vi "MeasBuilder Path.vi"(11 "error in (no error)":errorcluster) -> (4 "Template":path, 6 "Config":path, 8 "Python File":path, 15 "error out":errorcluster)   [LabVIEW 2021, in "Path Functions.lvlib"]
uses:
  Path Functions.lvlib
  <vilib>/Utility/sysdir.llb/System Directory Type.ctl
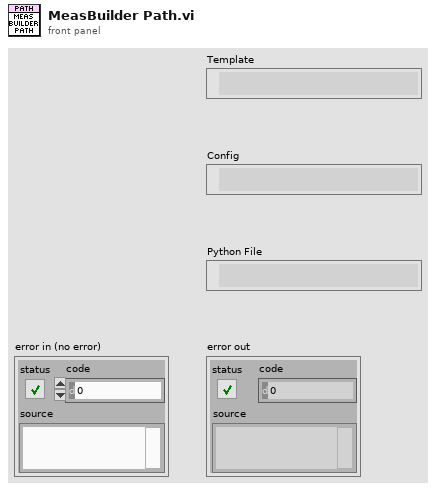
[diagram p1: front panel]
types:
  T1 = typedef "System Directory Type.ctl" = i32
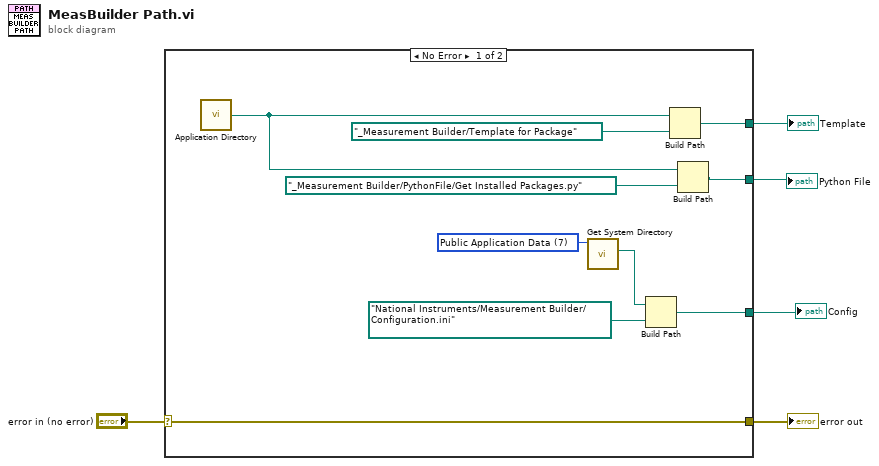
[diagram p0: block diagram]
diagram:
  n1 = case shown="No Error" "error in (no error)" {
    selector: "error in (no error)" -> [w13 w16]
    tunnel: [w14 _] -> w4
    tunnel: [w13 w16] -> w3
    tunnel: [w10 _] -> w2
    tunnel: [w6 _] -> w1
    frame No Error {
      w12 = T1 7 items=["User Home"=0, "User Desktop"=1, "User Documents"=2, "User Application Data"=3, "User Preferences"=4, "User Temporary"=5, "Public Documents"=6, "Public Application Data"=7, "Public Preferences"=8, "Public Cache"=13, "System Core Libraries"=9, "System Installed Libraries"=10, "Application Files"=11, "Boot Volume Root"=12] ("system directory type")
      n2 = call <vilib>:"Application Directory.vi"() -> ("Application Directory"=w7:path)
      n3 = call <vilib>:"Get System Directory.vi"("system directory type"=w12) -> ("system directory"=w11:path)  [unwired: 10 in]
      n4 = Build Path(base path=w11, name or relative path=path "National Instruments/Measurement Builder/Configuration.ini") -> (appended path=w10:path)
      n5 = Build Path(base path=w7, name or relative path=path "_Measurement Builder/Template for Package") -> (appended path=w14:path)
      n6 = Build Path(base path=w7, name or relative path=path "_Measurement Builder/PythonFile/Get Installed Packages.py") -> (appended path=w6:path)
    }
    frame Error {
    }
  }
  "error out" <- w3
  "Template" <- w4
  "Config" <- w2
  "Python File" <- w1
